vi "TestNewNamepathConversions.vi"() -> ()   [LabVIEW 2017]
uses:
  Mapper/ExposeMapperDataTypeEnum.ctl
  Mapper/ExposeObjectMapContainerTypeEnum.ctl
  Mapper/ExposeObjectMapNamepathData.ctl
  Mapper/ExposeMapperUpdateNamepathPartDescriptorEnum.ctl
  Mapper/ExposeMapperUpdateNamepathPartDescriptor.ctl
  Mapper/ExposeMapperObjectTypeEnum.ctl
  <vilib>/Utility/Data Type/Type Definitions/Data Type.ctl
  <vilib>/Utility/Data Type/NI_Data Type.lvlib
panel:
  in  "PositionConfig":T1={"UnitsToVolts"=0.005, "XToYRatio"=1.45, "InvertXY"=FALSE} caption="Positioner Config" {"XToYRatio" min=0.0; "UnitsToVolts" min=0.0 max=1.0}
  out "Array creation time":dbl
  out "Total Insert to value":dbl
  out "Total Make indo":dbl
  out "Flipper":bool
  in  "Ar":dbl[](array[numeric])
  out "Otype":T2[](array[typedef])
  in  "InitArSize":i32
  out "System Type":T3[](array[typedef])
  out "Container type":T4[](array[typedef])
  out "Values":variant[](array[variant])
  out "NPDsc":T5[](array[typedef])=[{"Parent Type"=enum."Invalid (Org. Val))", "Property Name"="", "Element Index"=0, "Control"=refnum, "Value Ref"=refnum, "Has value ref"=FALSE}] caption="Namepath Desription"
  in  "Namepath Info":T7={"Type"=enum."Real", "Value"=variant, "Namepath"="First@Num", "Container Type"=enum."Value"}
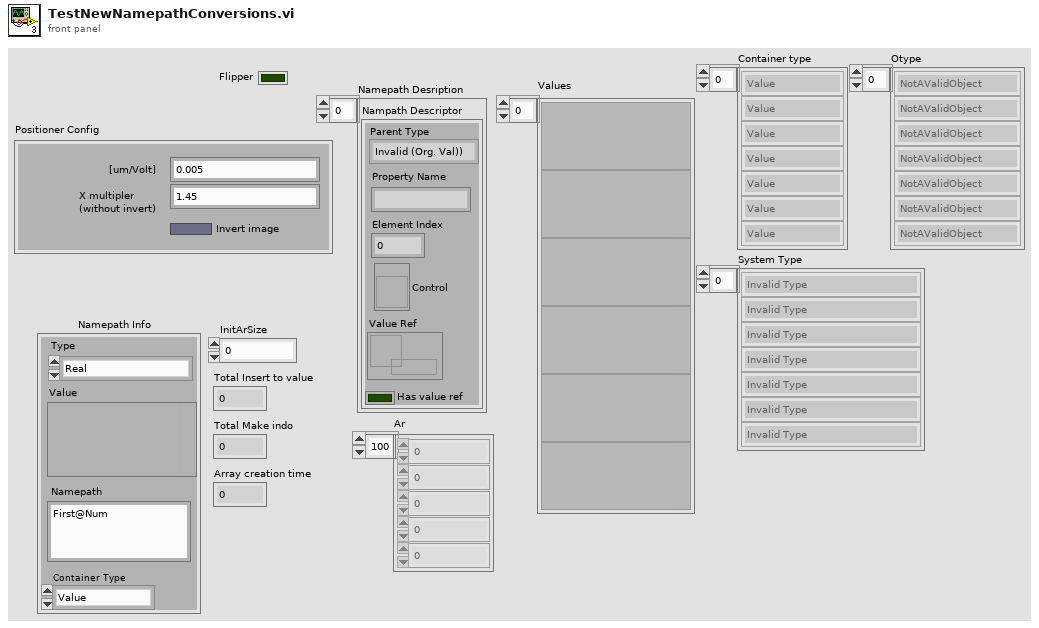
[diagram p1: front panel]
types:
  T1 = cluster{"UnitsToVolts":dbl, "XToYRatio":dbl, "InvertXY":bool}
  T2 = typedef "ExposeMapperObjectTypeEnum.ctl" = enum16{"NotAValidObject", "Value", "Variant", "Cluster", "Array", "Asng. Refnum"}
  T3 = typedef "NI_Data Type.lvlib/Data Type.ctl" = enum8{"Invalid Type", "Void", "I8", "I16", "I32", "I64", "U8", "U16", "U32", "U64", "Single Float", "Double Float", "Extended Float", "Single Complex", "Double Complex", "Extended Complex", "Enum U8", "Enum U16", "Enum U32", "Enum U64", "Single Float With Unit", "Double Float With Unit", "Extended Float With Unit", "Single Complex with Unit", "Double Complex with Unit", "Extended Complex with Unit", "Boolean", "String", "Path", "Picture", "Tag", "Array", "Cluster", "Variant", "LV Variant", "Waveform", "Timestamp", "Digital Waveform", "Digital Data", "ExpressData", "Refnum", "External Data", "VI", "Poly VI", "LabVIEW Class Instance", "Fixed Point"}
  T4 = typedef "ExposeObjectMapContainerTypeEnum.ctl" = enum16{"Value", "Array", "Waveform", "NetContainer"}
  T5 = typedef "ExposeMapperUpdateNamepathPartDescriptor.ctl" = cluster{"Parent Type":T6, "Property Name":string, "Element Index":i32, "Control":refnum<vi>, "Value Ref":refnum<data-value>, "Has value ref":bool}
  T6 = typedef "ExposeMapperUpdateNamepathPartDescriptorEnum.ctl" = enum16{"Invalid (Org. Val))", "Default Value", "Value", "Variant", "Cluster", "Array", "Refnum"}
  T7 = typedef "ExposeObjectMapNamepathData.ctl" = cluster{"Type":T8, "Value":variant, "Namepath":string, "Container Type":T4}
  T8 = typedef "ExposeMapperDataTypeEnum.ctl" = enum16{"NotData", "Real", "Complex", "String", "Boolean", "Container"}
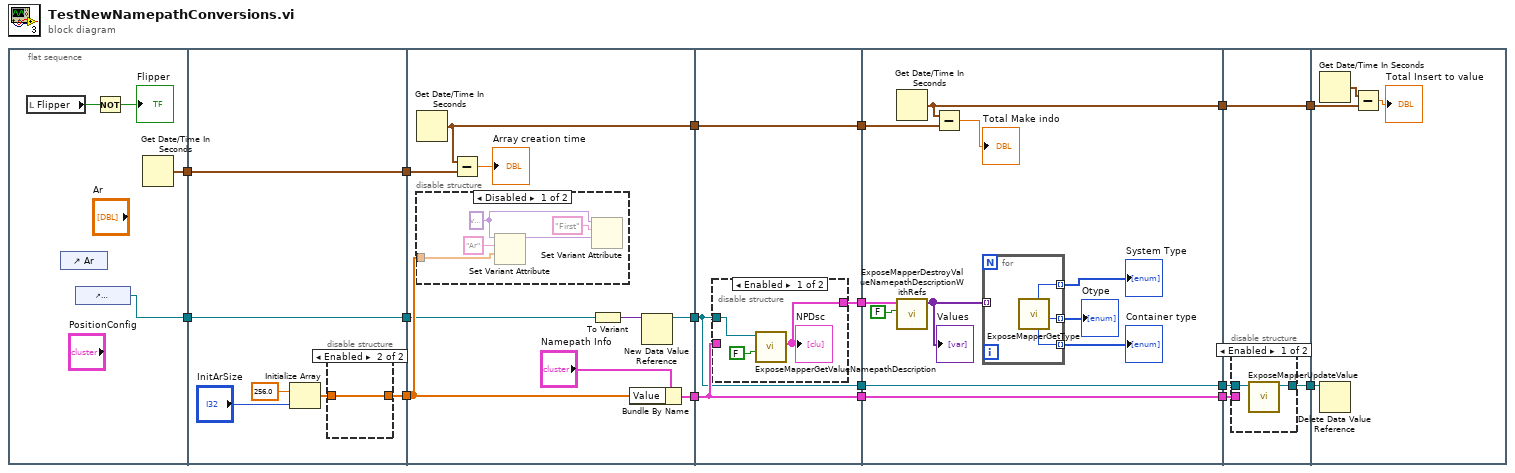
[diagram p0: block diagram]
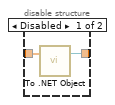
[diagram p2: hidden frame]
diagram:
  n1 = flat-sequence {
    tunnel: [w19] -> w3
    tunnel: [w18] -> w1
    tunnel: [w24] -> w5
    tunnel: [w23] -> w4
    tunnel: w3 -> [w23]
    tunnel: [w22] -> w2
    tunnel: w1 -> [w22]
    tunnel: [w38] -> w15
    tunnel: [w36] -> w13
    tunnel: [w34] -> w10
    tunnel: w5 -> [w35]
    tunnel: w4 -> [w33]
    tunnel: w2 -> [w31]
    tunnel: w15 -> [w48]
    tunnel: [w48] -> w14
    tunnel: w13 -> [w47]
    tunnel: [w47] -> w12
    tunnel: [w46] -> w11
    tunnel: w10 -> [w45]
    tunnel: [w45] -> w9
    tunnel: w14 -> [w62]
    tunnel: [w62] -> w17
    tunnel: w12 -> [w61]
    tunnel: [w61] -> w16
    tunnel: w11 -> [w60]
    tunnel: w9 -> [w54]
    tunnel: [w52] -> w7
    tunnel: w17 -> [w69]
    tunnel: w16 -> [w68]
    tunnel: [w67] -> w8
    tunnel: w7 -> [w66]
    tunnel: [w66] -> w6
    tunnel: w8 -> [w76]
    tunnel: w6 -> [w74]
    frame #0 {
      n2 = local read "Flipper"() -> (w21:bool)
      n3 = control-ref of="Ar"() -> ()  [unwired: 1 out]
      n4 = control-ref of="PositionConfig"() -> (w18:refnum<vi>)
      n5 = Not(x=w21) -> (.not. x?=→"Flipper":bool)
      n6 = Get Date/Time In Seconds() -> (seconds since 1Jan1904=w19:timestamp)
    }
    frame #1 {
      n7 = Initialize Array(256.0, "InitArSize") -> (w27:dbl[])
      n8 = disable-structure shown="Enabled" {
        disable-tunnel: w27 -> [w29 w30]
        disable-tunnel: [w28 w30] -> w24
        frame Disabled {
          n9 = call <vilib>:"To .NET Object.vi"("anything"=w29) -> (".NET object"=w28:refnum<k24>)  [unwired: 1 in, 1 out]
        }
        frame Enabled {
        }
      }
    }
    frame #2 {
      n10 = Get Date/Time In Seconds() -> (seconds since 1Jan1904=w34:timestamp)
      n11 = disable-structure shown="Disabled" {
        disable-tunnel: w35 -> [w44 _]
        frame Disabled {
          w41 = variant
          n12 = Set Variant Attribute(Variant=w41, name="Ar", value=w44) -> (Variant out=w43:variant)  [unwired: 1 in, 2 out]
          n13 = Set Variant Attribute(Variant=w41, name="First", value=w43) -> ()  [unwired: 1 in, 3 out]
        }
        frame Enabled {
        }
      }
      n14 = Subtract(x=w34, y=w33) -> (x-y=→"Array creation time":dbl)
      n15 = To Variant(anything=w31) -> (Variant=w37:variant)
      n16 = Bundle By Name(cluster="Namepath Info", "Value"=w35) -> (w38:T7)
      n17 = New Data Value Reference(data value=w37) -> (data value reference=w36:refnum<data-value>)  [unwired: 1 in, 1 out]
    }
    frame #3 {
      n18 = disable-structure shown="Enabled" {
        disable-tunnel: w48 -> [_ _]
        disable-tunnel: w47 -> [w51 _]
        disable-tunnel: [w49 _] -> w46
        frame Enabled {
          n19 = call "ExposeMapperGetValueNamepathDescription.vi"("ColRefVals"=FALSE, "Data Value Reference in"=w51) -> ("NPDsc"=w49:T5[])  [unwired: 7 in, 2 out]
          "NPDsc" <- w49
        }
        frame Disabled {
        }
      }
    }
    frame #4 {
      n20 = Get Date/Time In Seconds() -> (seconds since 1Jan1904=w52:timestamp)
      n21 = call "ExposeMapperDestroyValueNamepathDescriptionWithRefs.vi"("Collect values"=FALSE, "NPDsc"=w60) -> ("Values"=w58:variant[])  [unwired: 9 in]
      "Values" <- w58
      n22 = Subtract(x=w52, y=w54) -> (x-y=→"Total Make indo":dbl)
      n23 = for {
        tunnel: w58 -> [_] mode=indexing
        tunnel: [w65] -> w57 mode=indexing
        tunnel: [w64] -> w55 mode=indexing
        tunnel: [w63] -> w56 mode=indexing
        n24 = call "ExposeMapperGetType.vi"() -> ("OType"=w64:T2, "Container Type (Labview Value type)"=w65:T4, "System Type"=w63:T3)  [unwired: 6 in, 3 out]
      }
      "Container type" <- w57
      "System Type" <- w56
      "Otype" <- w55
    }
    frame #5 {
      n25 = disable-structure shown="Enabled" {
        disable-tunnel: w69 -> [_ _]
        disable-tunnel: w68 -> [w71 w72]
        disable-tunnel: [w70 w72] -> w67
        frame Enabled {
          n26 = call "ExposeMapperUpdateValue.vi"("Value In (or type, reference)"=w71) -> ("Value Out Ref"=w70:refnum<data-value>)  [unwired: 9 in, 1 out]
        }
        frame Disabled {
        }
      }
    }
    frame #6 {
      n27 = Get Date/Time In Seconds() -> (seconds since 1Jan1904=w75:timestamp)
      n28 = Delete Data Value Reference(data value reference=w76) -> ()  [unwired: 1 in, 2 out]
      n29 = Subtract(x=w75, y=w74) -> (x-y=→"Total Insert to value":dbl)
    }
  }
